vi "Complete Request.vi"(7 "Processing In":refnum<class "Processing.lvclass">, 11 "HTTPStatsHandler in":refnum<class "HTTPStatsHandler.lvclass">) -> (0 "error out":errorcluster, 5 "Processing":refnum<class "Processing.lvclass">)   [LabVIEW 2020, in "Vecto.lvlib" / "HTTPStatsHandler.lvclass"]
uses:
  HTTPStatsHandler.lvclass
  lv-http-server/HTTP Server/Processing/Processing.lvclass
  lv-http-server/HTTP Server/Processing/Processing.lvclass/Processing.ctl
  HTTPStatsHandler.lvclass/HTTPStatsHandler.ctl
  VectoService/VectoInfo.lvclass
  lv-http-util/HTTP Utils/Response/Response.lvclass
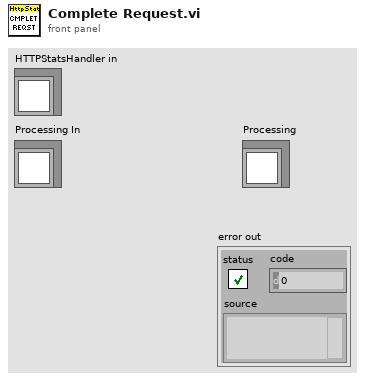
[diagram p1: front panel]
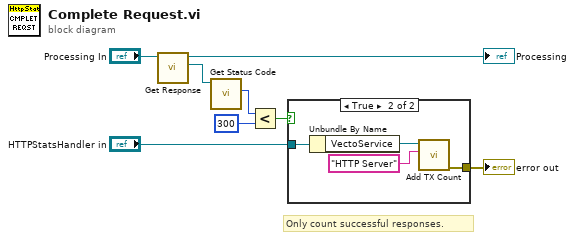
[diagram p0: block diagram]
diagram:
  # "Only count successful responses."
  n1 = call "Get Response.vi"("Processing in"="Processing In") -> ("Response"=w4:refnum<class "Response.lvclass">, "Processing out"=→"Processing":refnum<class "Processing.lvclass">)  [unwired: 9 in]
  n2 = call "Get Status Code.vi"("Response in"=w4) -> ("Status Code"=w3:u16)  [unwired: 8 in, 2 out]
  n3 = Less?(x=w3, y=u16 300) -> (x < y?=w1:bool)
  n4 = case shown="True" w1 {
    tunnel: "HTTPStatsHandler in" -> [_ w12]
    tunnel: [_ w9] -> w6
    frame False {
    }
    frame True {
      n5 = Unbundle By Name(w12) -> ("VectoService"=w11:refnum<class "VectoInfo.lvclass">)
      n6 = call "Add TX Count.vi"("Connection Name"="HTTP Server", "VectoService in"=w11) -> ("error out"=w9:errorcluster)  [unwired: 8 in, 1 out]
    }
  }
  "error out" <- w6
